vi "Wait Timer.vi"(8 "error in (no error)":errorcluster caption="错误输入（无错误）", 11 "Dely":u16(ring)=300 items=["10"=10, "20"=20, "50"=50, "80"=80, "100"=100, "200"=200, "300"=300, "400"=400, "500"=500, "600"=600, "700"=700, "800"=800, "900"=900, "1000"=1000]) -> (0 "error out":errorcluster caption="错误输出", 3 "毫秒计时值":u32)   [LabVIEW 2014]
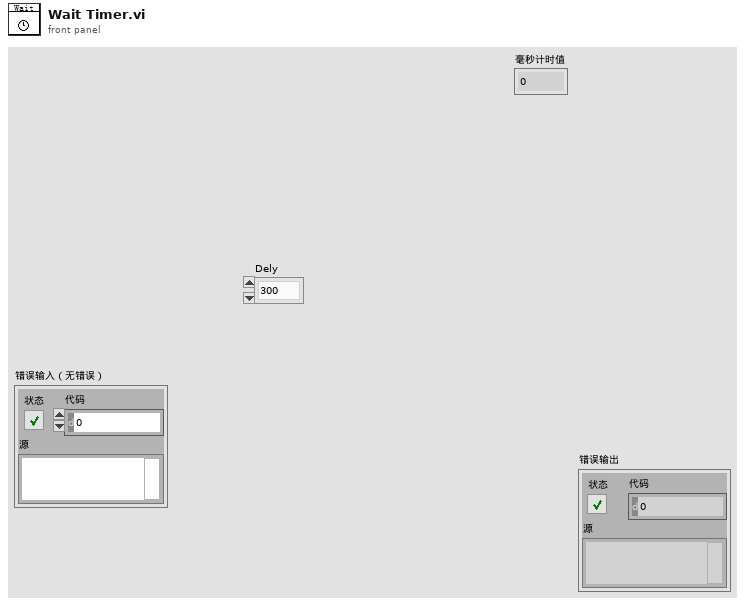
[diagram p1: front panel]
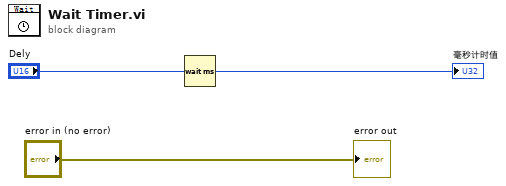
[diagram p0: block diagram]
diagram:
  n1 = Wait (ms)(milliseconds to wait="Dely") -> (millisecond timer value=→"毫秒计时值":u32)
  "error out" <- "error in (no error)"
